vi "DCA Execute Test.vi"(5 "Attenuation Calculation":enum32{"Power", "Voltage"}(ring), 6 "Driver Refs":T9, 7 "Colors":cluster{"Pass":u32, "Fail":u32, "Nop":u32}={"Pass"=6618880, "Fail"=16711680, "Nop"=16777226}, 8 "error in (no error)":errorcluster, 9 "Test Parameters In":T11={"Stimulus"={"Use Instrument"=FALSE, "Normalize"=FALSE, "Blank Screen"=FALSE, "Measurement Type"=enum."Voltage DC", "Range"=enum."Auto", "Resolution"=enum."Auto"}, "Measurement"={"Topology"=enum."PI-Network", "Lock Topology"=FALSE, "ATTN Calc"=enum."Power", "Zo"=50.0}, "Limits"=[], "Normalization"={"Normalized?"=FALSE, "Rab Value"=0.0, "Rac Value"=0.0, "Rbc Value"=0.0}}, 10 "Topology":T6, 11 "Limit Status Ref":refnum<vi>) -> (0 "error out":errorcluster, 1 "Test Parameters Out":T11={"Stimulus"={"Use Instrument"=FALSE, "Normalize"=FALSE, "Blank Screen"=FALSE, "Measurement Type"=enum."Voltage DC", "Range"=enum."Auto", "Resolution"=enum."Auto"}, "Measurement"={"Topology"=enum."PI-Network", "Lock Topology"=FALSE, "ATTN Calc"=enum."Power", "Zo"=50.0}, "Limits"=[], "Normalization"={"Normalized?"=FALSE, "Rab Value"=0.0, "Rac Value"=0.0, "Rbc Value"=0.0}}, 2 "Passed?":bool, 3 "Measurement Values":T10, 4 "Limits and Passed?":cluster{"Limits":T1[], "Passed? Array":bool[]})   [LabVIEW 2011]
uses:
  TypeDefs/DCA Test Parameters.ctl
  TypeDefs/DCA Stimulus Parameters.ctl
  TypeDefs/DCA Measurement Cluster.ctl
  TypeDefs/DCA Topology.ctl
  TypeDefs/DCA Attenuation Calculation.ctl
  TypeDefs/DCA Limit.ctl
  TypeDefs/DCA Limit Quantity.ctl
  TypeDefs/DCA Limit Comparison.ctl
  TypeDefs/DCA Limit Operation.ctl
  Test Referential Limit.ctl
  TypeDefs/DCA Calibration State.ctl
  drivers/DMM/DMM Driver Ref.ctl
  drivers/SWI/SWI Driver Ref.ctl
  TypeDefs/DCA Measurement Values.ctl
  TypeDefs/DCA Measurement.ctl
  drivers/SWI/SWI Command.ctl
  drivers/DMM/DMM Command.ctl
panel:
  out "dup Driver Refs":T9
  in  "Empty Measurement Values":T10
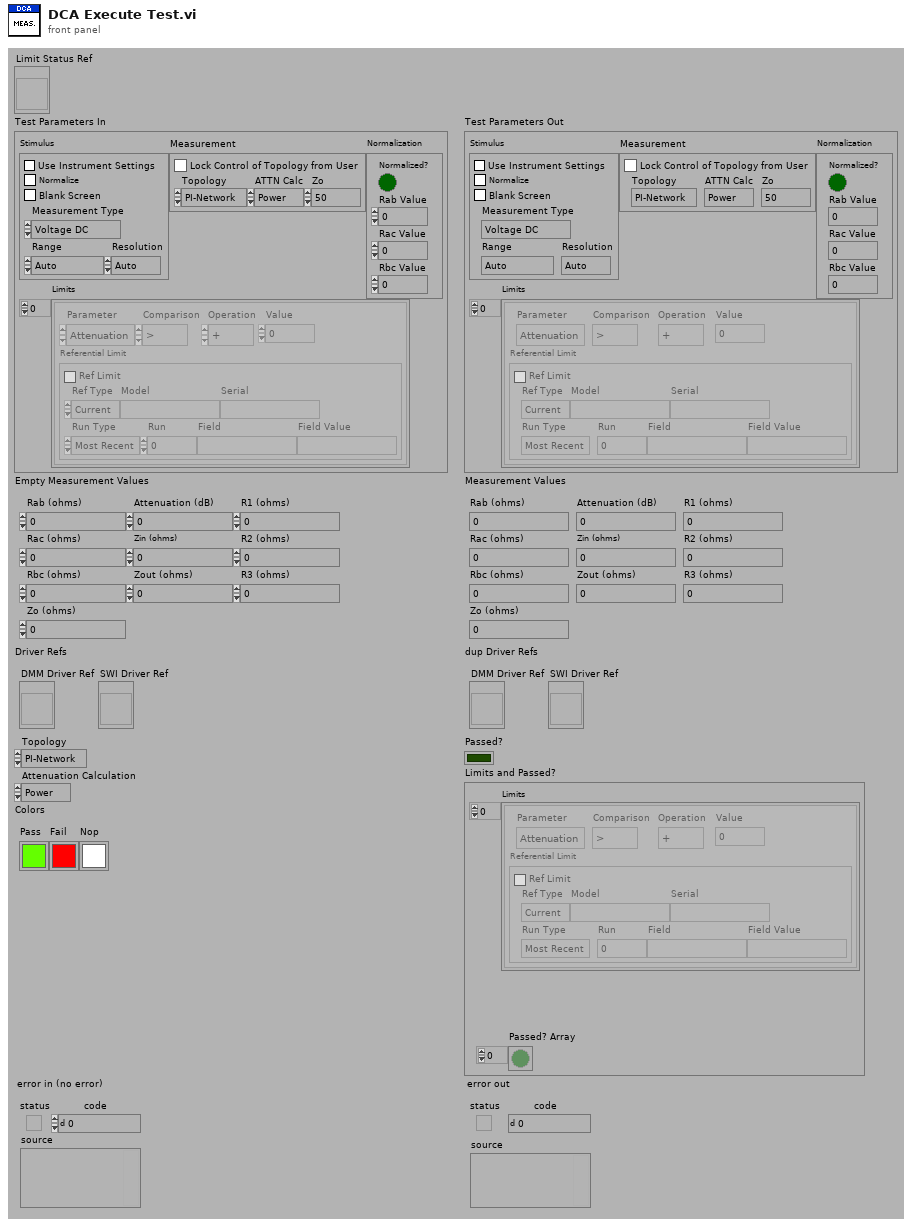
[diagram p1: front panel]
types:
  T1 = typedef "DCA Limit.ctl" = cluster{"Parameter":T2, "Comparison":T3, "Operation":T4, "Value":dbl, "Referential Limit":T5}
  T2 = typedef "DCA Limit Quantity.ctl" = enum16{"Attenuation", "Zin", "Zout", "R1", "R2", "R3", "Rab", "Rac", "Rbc"}
  T3 = typedef "DCA Limit Comparison.ctl" = enum16{">", ">=", "<", "<="}
  T4 = typedef "DCA Limit Operation.ctl" = enum16{"+", "-"}
  T5 = typedef "Test Referential Limit.ctl" = cluster{"Ref Limit":bool, "Ref Type":enum16{"Current", "Specify"}, "Model":string, "Serial":string, "Run Type":enum16{"Most Recent", "Run #", "Match Field"}, "Run":i32, "Field":string, "Field Value":string}
  T6 = typedef "DCA Topology.ctl" = enum32{"PI-Network", "T-Network"}
  T7 = typedef "DMM Driver Ref.ctl" = refnum<vi>
  T8 = typedef "SWI Driver Ref.ctl" = refnum<vi>
  T9 = cluster{"DMM Driver Ref":T7, "SWI Driver Ref":T8}
  T10 = typedef "DCA Measurement Values.ctl" = cluster{"Rab (ohms)":dbl, "Rac (ohms)":dbl, "Rbc (ohms)":dbl, "Zo (ohms)":dbl, "Attenuation (dB)":dbl, "Zin (ohms)":dbl, "Zout (ohms)":dbl, "R1 (ohms)":dbl, "R2 (ohms)":dbl, "R3 (ohms)":dbl}
  T11 = typedef "DCA Test Parameters.ctl" = cluster{"Stimulus":T12, "Measurement":T13, "Limits":T1[], "Normalization":T15}
  T12 = typedef "DCA Stimulus Parameters.ctl" = cluster{"Use Instrument":bool, "Normalize":bool, "Blank Screen":bool, "Measurement Type":enum16{"Voltage DC", "Voltage DC Ratio", "Voltage AC", "Current DC", "Current AC", "Resistance", "Fresistance", "Frequency", "Period", "Continuity", "Diode"}, "Range":enum16{"Auto", "Minimum", "Maximum", "100", "1,000", "10,000", "100,000", "1,000,000", "10,000,000", "100,000,000"}, "Resolution":enum16{"Auto", "4 1/2", "5 1/2", "6 1/2"}}
  T13 = typedef "DCA Measurement Cluster.ctl" = cluster{"Topology":T6, "Lock Topology":bool, "ATTN Calc":T14, "Zo":dbl}
  T14 = typedef "DCA Attenuation Calculation.ctl" = enum32{"Power", "Voltage"}
  T15 = typedef "DCA Calibration State.ctl" = cluster{"Normalized?":bool, "Rab Value":dbl, "Rac Value":dbl, "Rbc Value":dbl}
  T16 = typedef "DCA Measurement.ctl" = enum16{"Rab", "Rac", "Rbc"}
  T17 = typedef "SWI Command.ctl" = enum16{"LOAD", "INITIALIZE", "PRESET", "SET STIMULUS", "GET STIMULUS", "GET INFO", "RELEASE", "UNLOAD"}
  T18 = typedef "DMM Command.ctl" = enum16{"LOAD", "INITIALIZE", "PRESET", "GET STIMULUS", "SET STIMULUS", "MEASURE", "RELEASE", "UNLOAD", "GET CALIBRATION", "CALIBRATE"}
  T19 = typedef "Sea-Level SWI Position.ctl" = cluster{"Port 1 (0)":cluster{"0":bool, "1":bool, "2":bool, "3":bool, "4":bool, "5":bool, "6":bool, "7":bool}, "Port 2 (1)":cluster{"0":bool, "1":bool, "2":bool, "3":bool, "4":bool, "5":bool, "6":bool, "7":bool}, "Port 3 (2)":cluster{"0":bool, "1":bool, "2":bool, "3":bool, "4":bool, "5":bool, "6":bool, "7":bool}, "Port 4 (3)":cluster{"0":bool, "1":bool, "2":bool, "3":bool, "4":bool, "5":bool, "6":bool, "7":bool}}
  T20 = typedef "DMM Measurement.ctl" = dbl
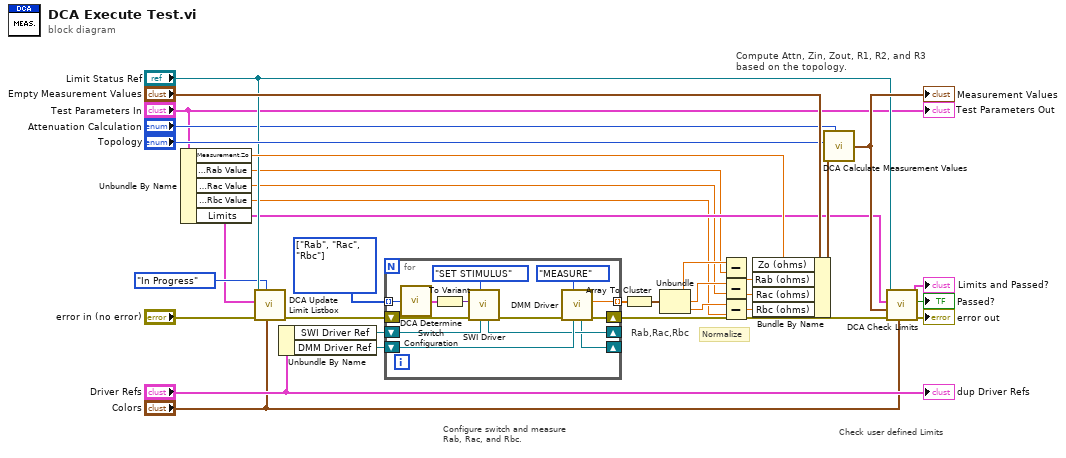
[diagram p0: block diagram]
diagram:
  w30 = T16[] [enum."Rab", enum."Rac", enum."Rbc"] items=["Rab", "Rac", "Rbc"]
  # "Normalize"
  # "Compute Attn, Zin, Zout, R1, R2, and R3\nbased on the topology."
  # "Check user defined Limits"
  # "Configure switch and measure\nRab, Rac, and Rbc."
  # "Rab,Rac,Rbc"
  n1 = Unbundle By Name("Test Parameters In") -> ("Measurement.Zo"=w24:dbl, "Normalization.Rab Value"=w3:dbl, "Normalization.Rac Value"=w2:dbl, "Normalization.Rbc Value"=w1:dbl, "Limits"=w10:T1[])
  n2 = call "DCA Update Limit Listbox.vi"("Colors"="Colors", "State (Pass/Fail)"=enum16{"Reset", "In Progress", "Pass/Fail"}."In Progress", "error in (no error)"="error in (no error)", "Limits"=w10, "Limit Status Ref"="Limit Status Ref") -> ("error out"=w17:errorcluster)  [unwired: 1 in, 5 out]
  n3 = Unbundle By Name("Driver Refs") -> ("SWI Driver Ref"=w32:T8, "DMM Driver Ref"=w31:T7)
  n4 = for {
    tunnel: w30 -> [w38] mode=indexing
    tunnel: [w37] -> w28 mode=indexing
    shift-right: [w36] -> w20
    shift-left: w17 -> [w43]
    shift-right: [w34] -> _
    shift-left: w31 -> [w40]
    shift-right: [w35] -> _
    shift-left: w32 -> [w41]
    n5 = call "DCA Determine Switch Configuration.vi"("Measurement"=w38) -> ("SWI Position"=w39:T19)
    n6 = To Variant(anything=w39) -> (Variant=w33:variant)
    n7 = call "SWI Driver.vi"("Drv Refnum"=w41, "SWI Command"=SWI_Command."SET STIMULUS", "error in (no error)"=w43, "SWI Position In"=w33) -> ("error out"=w42:errorcluster, "dup Drv Refnum"=w35:T8)  [unwired: 1 in, 5 out]
    n8 = call "DMM Driver.vi"("Drv Refnum"=w40, "DMM Command"=DMM_Command."MEASURE", "error in (no error)"=w42) -> ("error out"=w36:errorcluster, "DMM Measurement"=w37:T20, "dup Drv Refnum"=w34:T7)  [unwired: 2 in, 4 out]
  }
  n9 = Array To Cluster(array=w28) -> (cluster=w27:cluster{"[0]":T20, "[1]":T20, "[2]":T20})
  n10 = Unbundle(w27) -> ("[0]"=w8:T20, "[1]"=w4:T20, "[2]"=w6:T20)
  n11 = Subtract(x=w8, y=w3) -> (x-y=w9:T20)
  n12 = Subtract(x=w4, y=w2) -> (x-y=w5:T20)
  n13 = Subtract(x=w6, y=w1) -> (x-y=w7:T20)
  n14 = Bundle By Name(cluster="Empty Measurement Values", "Zo (ohms)"=w24, "Rab (ohms)"=w9, "Rac (ohms)"=w5, "Rbc (ohms)"=w7) -> (w26:T10)
  n15 = call "DCA Calculate Measurement Values.vi"("Topology"="Topology", "Measurement Values"=w26, "Attenuation Calculation"="Attenuation Calculation") -> ("Calculated Measurement Values"=w22:T10)  [unwired: 2 out]
  "Measurement Values" <- w22
  n16 = call "DCA Check Limits.vi"("Colors"="Colors", "error in (no error)"=w20, "Measurement Values"=w22, "Limits"=w10, "Limit Status Ref"="Limit Status Ref") -> ("error out"=→"error out":errorcluster, "Passed?"=→"Passed?":bool, "Limits and Passed?"=→"Limits and Passed?":cluster{"Limits":T1[], "Passed? Array":bool[]})  [unwired: 4 out]
  "Test Parameters Out" <- "Test Parameters In"
  "dup Driver Refs" <- "Driver Refs"
